vi "Main.vi"() -> ()   [LabVIEW 2013]
doc: "This Continuous Measurement sample project is based on the Queued Message Handler template.\n\nThe Event Handling Loop generates messages based on user interface actions.\n\nThe Message Handling Loop processes messages generated by the Event Handling Loop, or by other messages. There are also Acquisition and Logging message handling loop subVIs, and a chart updating loop."
uses:
  Settings/Settings.ctl
  Logging/Logging Configuration.ctl
  Piezo/Hardware Configuration.ctl
  Capacitive/Hardware Configuration.ctl
  Acquisition/Hardware Configuration.ctl
  Acquisition/Counter Configuration.ctl
  ADC/ADC Configuration.ctl
  controls/UI Data.ctl
  controls/UI State.ctl
  support/Message Queue/Enqueue Message (Single).vi
  <vilib>/measure/madcrms.llb/Averaged DC-RMS for 1 Chan.vi
  <vilib>/Utility/error.llb/Error Cluster From Error Code.vi
  <vilib>/ErrorRing/Error Ring.xnode
  Acquisition/Acquisition.lvlib
  Logging/Logging.lvlib
  Settings/Settings.lvlib
  support/User Event - Stop/User Event - Stop.lvlib
  support/Message Queue/Message Queue.lvlib
  <vilib>/ptbypt/NI_PtbyPt.lvlib
  Piezo/Piezo.lvlib
  Feedback/Feedback.lvlib
  <vilib>/measure/NI_MAPro.lvlib
  XY/XY.lvlib
  support/Data Notifiers/Data Notifiers.lvlib
  Capacitive/Capacitive.lvlib
panel:
  in  "Feedback Settings":T1={"Setpoint (cnt)"=10.0, "Refresh Time (s)"=1.0, "K_p (nm/cnt)"=0.3, "Averaging Time"=1.0, "T_i (s)"=0.3, "T_d (s)"=1.0, "Error Signal Source"=0} {"Error Signal Source" items=["External Input", "APD Signal"]}
  in  "Scan!":bool
  in  "Auto \nFB On":bool
  out "Control Status":string
  in  "Averaging Time (s)":dbl=3.0
  in  "Average and send\nto Setpoint":bool
  out "average":dbl
  in  "averaging time":dbl=1000.0 format="%#_13g"
  out "Cap Readout":sgl
  out "Cap Status":string
  in  "Enable Sensor":bool
  out "Status 4":string
  in  "initialize":bool
  in  "PSD points":i32=1000
  out "Status 3":string
  out "Y":sgl
  out "X":sgl
  in  "Next Button":bool
  in  "Up Button":bool
  in  "Down Button":bool
  in  "Previous Button":bool
  in  "Jog Speed":u16(ring) items=["0", "1", "2", "3"]
  in  "Enable XY":bool
  out "Status":bool
  in  "Settings 3":bool
  in  "Stop 2":bool
  in  "Start 2":bool
  in  "Settings 2":bool
  in  "Enable Feedback!":bool
  in  "Scan Settings":T2={"Dwell Time (s)"=1.0, "Max Height"=10.0, "Min Height"=9.0, "Step Size (um)"=0.01}
  in  "Start Saving":bool
  out "PiezoPosition":sgl
  out "Lag!! (unconnected)":bool
  out "Scan Duration: (s)":dbl
  in  "Do move":bool
  in  "Move to (um)":sgl
  out "PSD":dbl[](graph)
  out "Data":dbl[][](graph)
  in  "Settings":bool
  in  "Start":bool
  in  "Stop":bool
  out "Status":string
  in  "Exit":bool
  # "Recording"
  # "Position Control"
  # "Acquisition"
  # "Piezo Controller"
  # "X-Y Stage"
  # "Displacement Sensor"
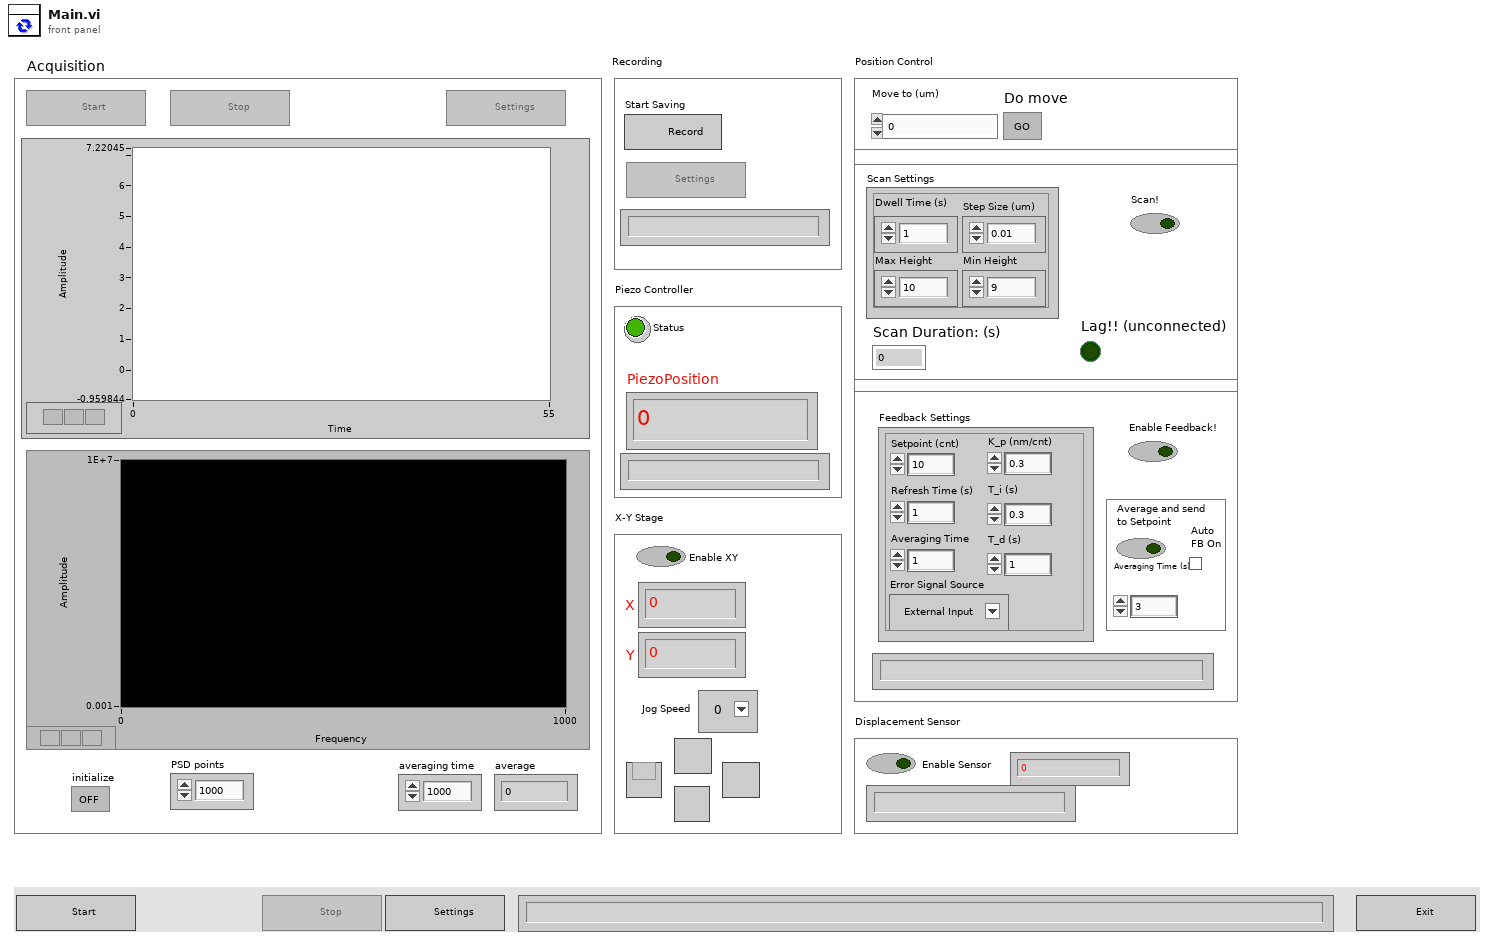
[diagram p1: front panel]
types:
  T1 = cluster{"Setpoint (cnt)":dbl, "Refresh Time (s)":dbl, "K_p (nm/cnt)":dbl, "Averaging Time":dbl, "T_i (s)":dbl, "T_d (s)":dbl, "Error Signal Source":u16}
  T2 = cluster{"Dwell Time (s)":dbl, "Max Height":dbl, "Min Height":dbl, "Step Size (um)":dbl}
  T3 = typedef "UI State.ctl" = cluster{"UI State":enum16{"Idle", "Acquiring and Logging", "Waiting for Exit", "Waiting for Stop"}, "Acq On":bool, "Log On":bool, "Piezo On":bool, "XY On":bool, "Cap On":bool}
  T4 = typedef "UI Data.ctl" = cluster{"Start Ref":refnum<vi>, "Trigger Ref":refnum<vi>, "Stop Ref":refnum<vi>, "Settings Ref":refnum<vi>, "Status Ref":refnum<vi>, "Exit Ref":refnum<vi>, "Data Ref":refnum<vi>, "Record Ref":refnum<vi>}
  T5 = typedef "Settings.lvlib/Settings.ctl" = cluster{"Logging Configuration":T6, "Piezo Config":T7, "Capacitive Config":T8, "Hardware Config":T9}
  T6 = typedef "Logging.lvlib/Logging Configuration.ctl" = cluster{"Log File Base Path":path, "Max Samples":u32, "File Refnum":refnum<file>, "Log Piezo":bool, "Piezo File Refnum":refnum<file>}
  T7 = typedef "Piezo.lvlib/Hardware Configuration.ctl" = cluster{"Piezo Serial Number":i32, "MG17Piezo":refnum<k7>, "Setpoint (um)":sgl}
  T8 = typedef "Capacitive.lvlib/Hardware Configuration.ctl" = cluster{"IP Address":string, "Handle":u32, "Refresh Time (ms)":dbl}
  T9 = typedef "Acquisition.lvlib/Hardware Configuration.ctl" = cluster{"Data Source":u16, "Counter Configuration":T10, "ADC Configuration":T11}
  T10 = typedef "Acquisition.lvlib/Counter Configuration.ctl" = cluster{"DAQmx Task":refnum<k21>, "Counter(s)":tag, "samples per readout":i32}
  T11 = typedef "Acquisition.lvlib/ADC Configuration.ctl" = cluster{"DAQmx Task":refnum<k21>, "Channel(s)":tag, "samples per readout":i32, "Sample Rate (s/s)":i32, "Max Voltage":dbl, "Min Voltage":dbl}
  T12 = typedef "Data Notifiers.lvlib/All Data Notifiers.ctl" = cluster{"APD Data Notifier":refnum<notifier>, "Piezo Readout Notifier":refnum<notifier>, "XY Readout Notifier":refnum<notifier>, "Capacitive Readout Notifier":refnum<notifier>}
  T13 = typedef "Message Queue.lvlib/All Message Queues.ctl" = cluster{"UI":refnum<queue>, "Acquisition":refnum<queue>, "Logging":refnum<queue>, "Piezo":refnum<queue>, "Feedback":refnum<queue>, "XY":refnum<queue>, "Capacitive":refnum<queue>}
  T14 = enum16{"Idle", "Acquiring and Logging", "Waiting for Exit", "Waiting for Stop"}
  T15 = enum8{"Enabled", "Disabled", "Disabled and Grayed Out"}
  T16 = typedef "Acquisition.lvlib/APD Notifier Cluster.ctl" = cluster{"data":dbl[][], "t0":i32}
  T17 = typedef "XY.lvlib/XY Display.ctl" = cluster{"X Position":sgl, "Y Position":sgl}
  T18 = typedef "Piezo.lvlib/Piezo display.ctl" = cluster{"PiezoPosition":sgl, "Counter Time":i32}
  T19 = typedef "Capacitive.lvlib/Capacitive Signal Cluster.ctl" = cluster{"Readout":sgl, "Time":i32}
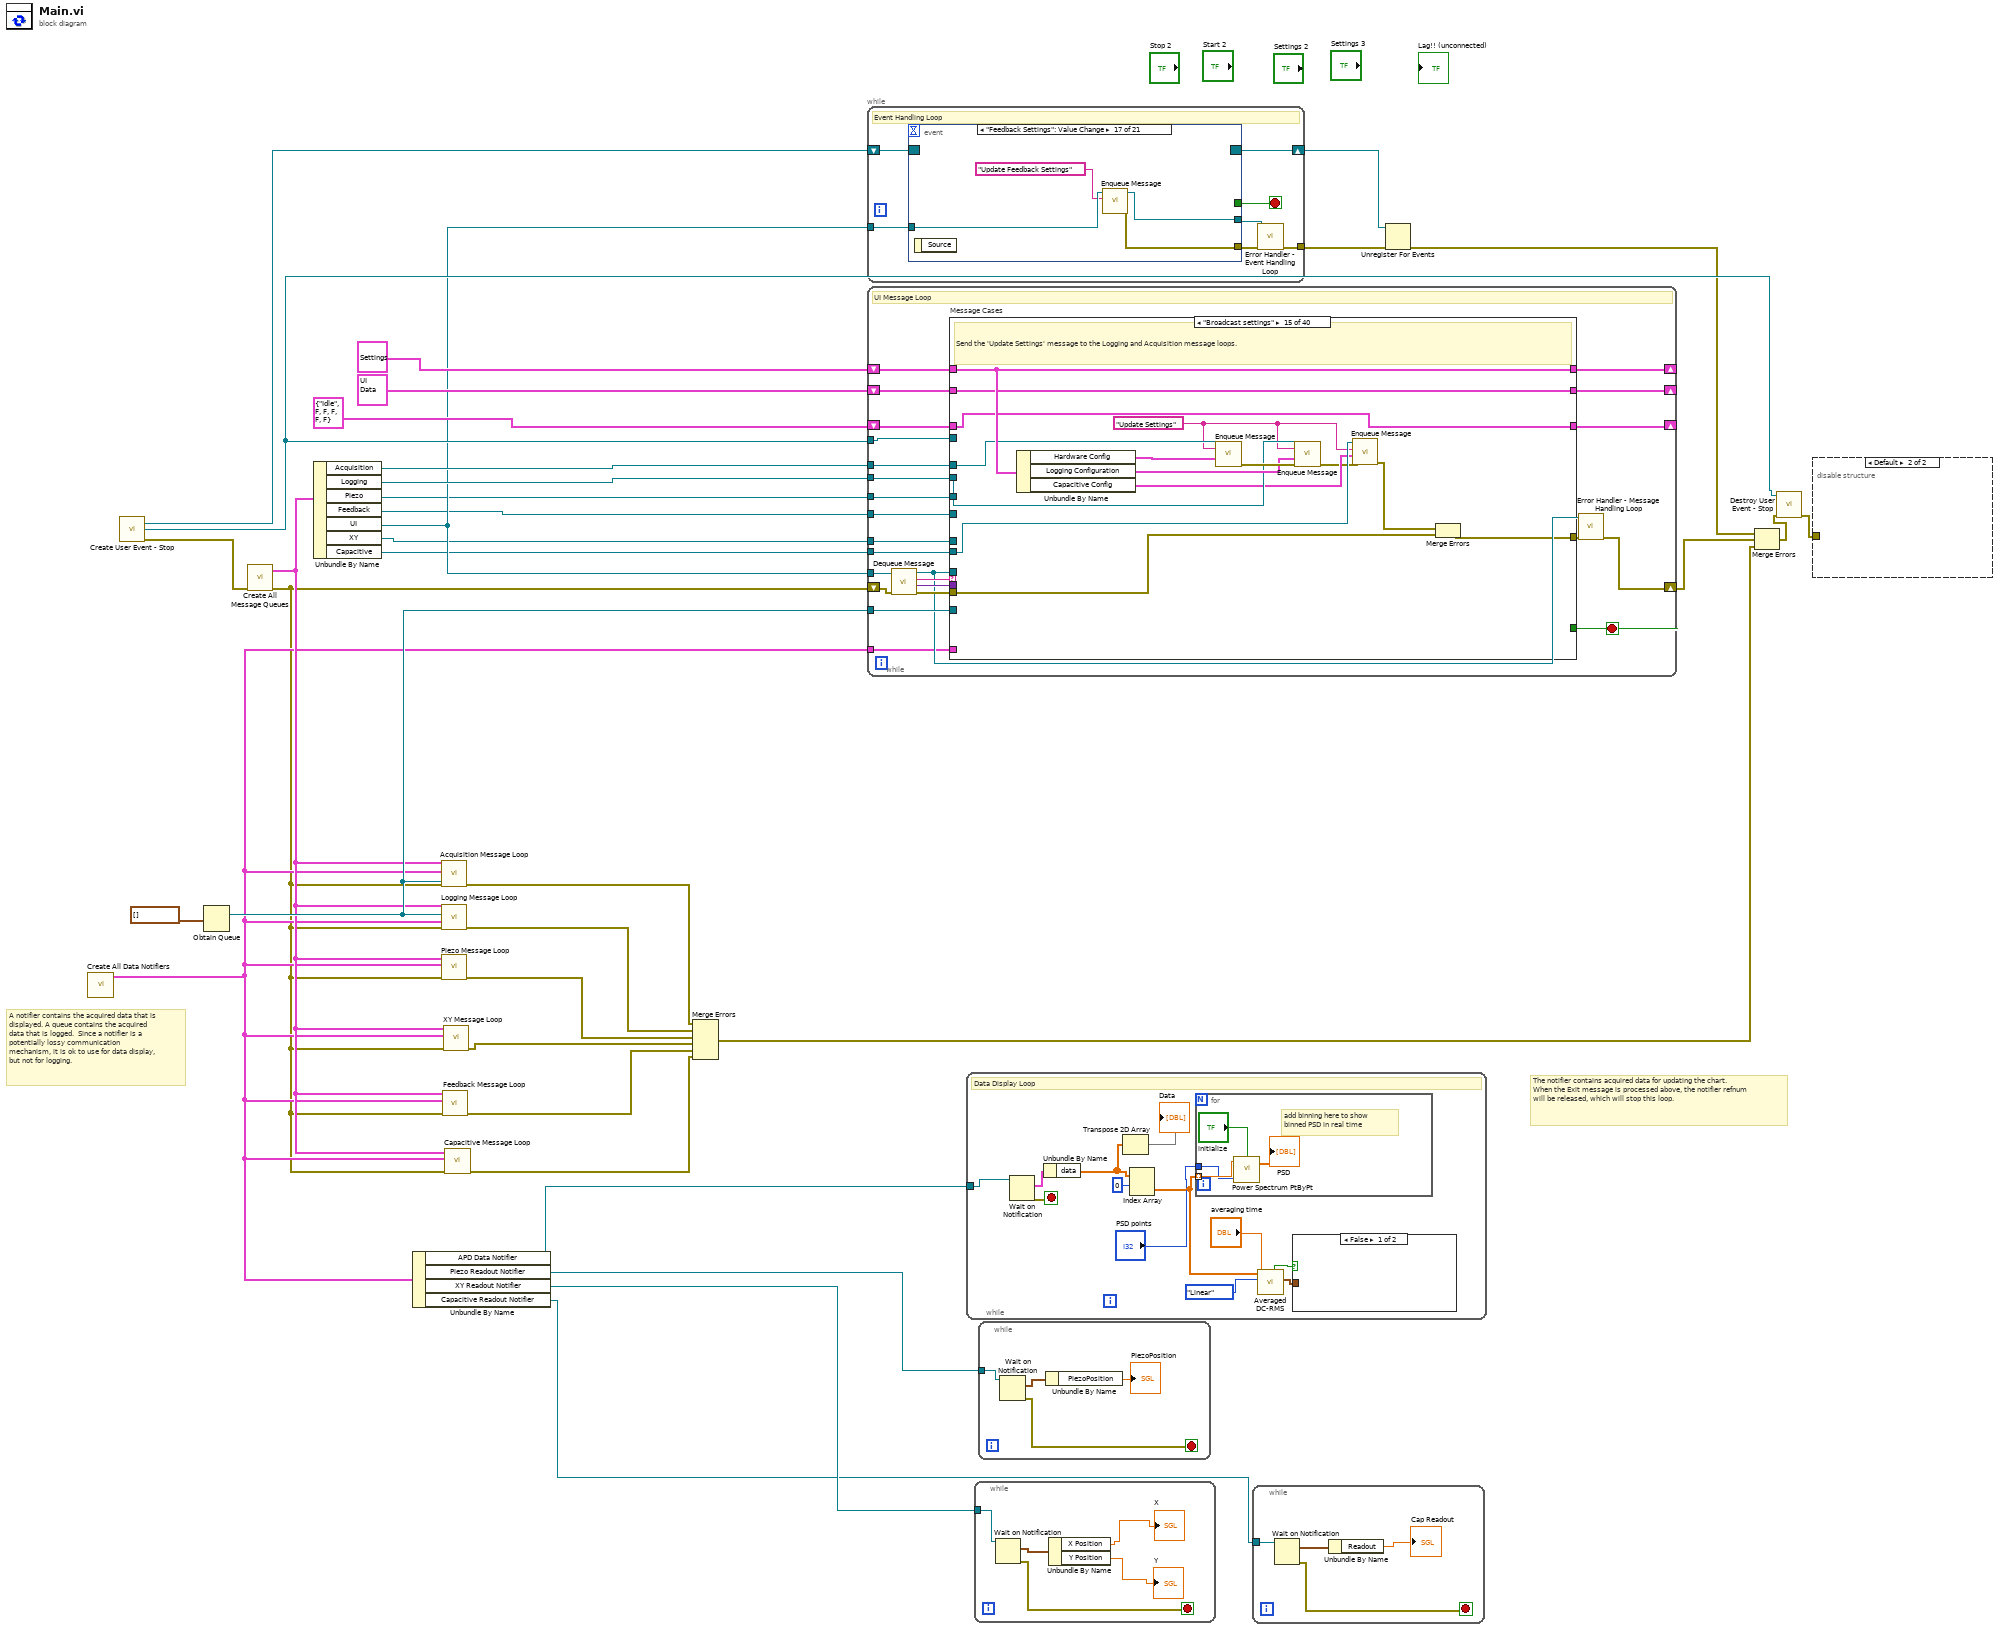
[diagram p0: block diagram]
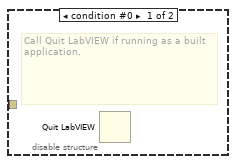
[diagram p2: hidden frame]
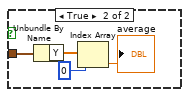
[diagram p3: hidden frame]
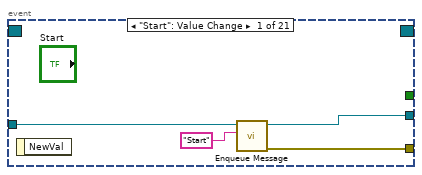
[diagram p4: hidden frame]
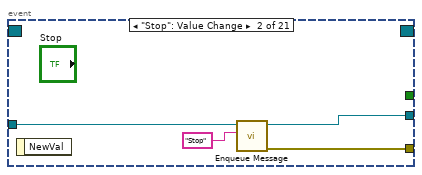
[diagram p5: hidden frame]
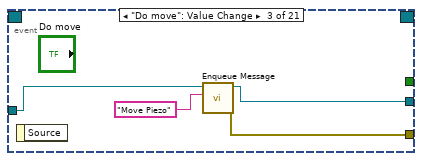
[diagram p6: hidden frame]
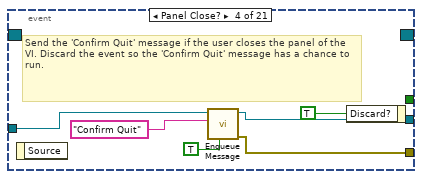
[diagram p7: hidden frame]
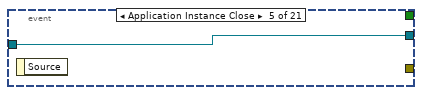
[diagram p8: hidden frame]
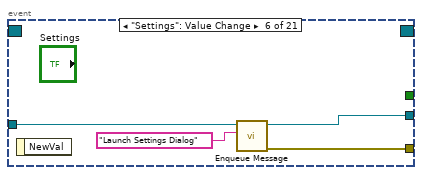
[diagram p9: hidden frame]
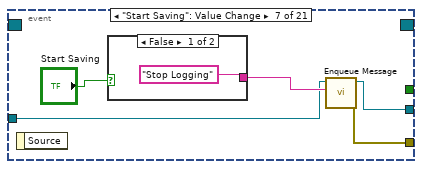
[diagram p10: hidden frame]
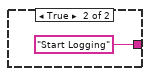
[diagram p11: hidden frame]
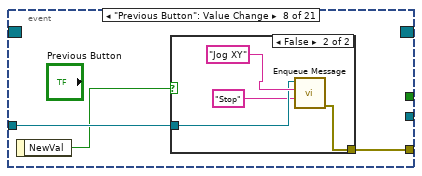
[diagram p12: hidden frame]
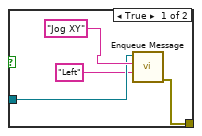
[diagram p13: hidden frame]
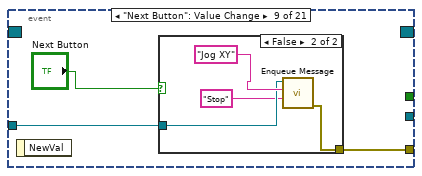
[diagram p14: hidden frame]
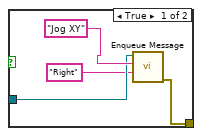
[diagram p15: hidden frame]
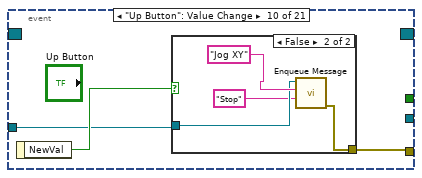
[diagram p16: hidden frame]
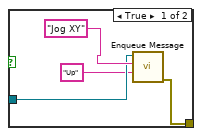
[diagram p17: hidden frame]
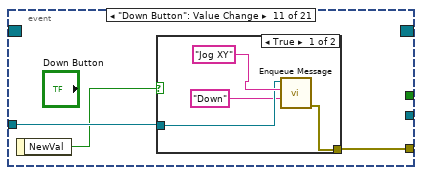
[diagram p18: hidden frame]
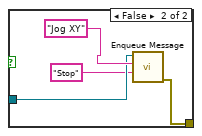
[diagram p19: hidden frame]
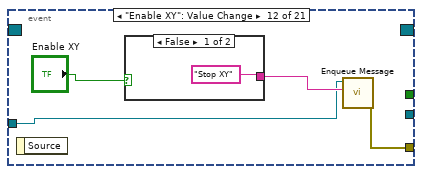
[diagram p20: hidden frame]
diagram:
  # "A notifier contains the acquired data that is displayed. A queue contains the acquired data that is logged.  Since a notifier is a potentially lossy communication mechanism, it is ok to use for data display, but not for logging."
  # "The notifier contains acquired data for updating the chart. When the Exit message is processed above, the notifier refnum will be released, which will stop this loop."
  n1 = call "Create All Data Notifiers.vi"() -> ("Initialized Data Notifiers"=w10:T12)  [unwired: 11 in]
  n2 = call "Create User Event - Stop.vi"() -> ("error out"=w30:errorcluster, "User Event - Stop"=w31:refnum<user-event>, "Stop Event Registration Refnum"=w32:refnum<event-registration>)  [unwired: 9 in]
  n3 = Obtain Queue(element data type=waveform(dbl)[] []) -> (queue out=w22:refnum<queue>)  [unwired: 4 in, 2 out]
  n4 = call "Create All Message Queues.vi"("error in (no error)"=w30) -> ("error out"=w9:errorcluster, "Message Queues out"=w11:T13)  [unwired: 9 in]
  n5 = Unbundle By Name(w11) -> ("Acquisition"=w25:refnum<queue>, "Logging"=w24:refnum<queue>, "Piezo"=w18:refnum<queue>, "Feedback"=w17:refnum<queue>, "UI"=w19:refnum<queue>, "XY"=w16:refnum<queue>, "Capacitive"=w12:refnum<queue>)
  n6 = Unbundle By Name(w10) -> ("APD Data Notifier"=w15:refnum<notifier>, "Piezo Readout Notifier"=w14:refnum<notifier>, "XY Readout Notifier"=w13:refnum<notifier>, "Capacitive Readout Notifier"=w1:refnum<notifier>)
  n7 = call "Acquisition Message Loop.vi"("error in (no error)"=w9, "Data Queue"=w22, "Data Notifiers"=w10, "Message Queues"=w11) -> ("error out"=w5:errorcluster)  [unwired: 7 in]
  n8 = call "Logging Message Loop.vi"("error in (no error)"=w9, "Data Notifiers"=w10, "Data Queue"=w22, "Message Queues"=w11) -> ("error out"=w6:errorcluster)  [unwired: 7 in]
  n9 = call "Piezo Message Loop.vi"("error in (no error)"=w9, "Data Notifiers"=w10, "Message Queues"=w11) -> ("error out"=w7:errorcluster)  [unwired: 8 in]
  n10 = call "Feedback Message Loop.vi"("error in (no error)"=w9, "Data Notifiers"=w10, "Message Queues"=w11) -> ("error out"=w4:errorcluster)  [unwired: 8 in]
  n11 = call "XY Message Loop.vi"("error in (no error)"=w9, "Data Notifiers"=w10, "Message Queues"=w11) -> ("error out"=w8:errorcluster)  [unwired: 8 in]
  n12 = call "Capacitive Message Loop.vi"("error in (no error)"=w9, "Data Notifiers"=w10, "Message Queues"=w11) -> ("error out"=w3:errorcluster)  [unwired: 8 in]
  n13 = Merge Errors(w5, w6, w7, w8, w4, w3) -> (w2:errorcluster)
  n14 = while {
    tunnel: w19 -> [w41]
    tunnel: [w36] -> w34
    shift-right: [w40] -> w27
    shift-left: w32 -> [w42]
    stop <- w39 stop-if-true
    # "Event Handling Loop"
    n15 = event shown="[16] \"Feedback Settings\": Value Change" {
      selector: w42 -> [_ _ _ _ _ _ _ _ _ _ _ _ _ _ _ _ _ _ _ _ _]
      dyn-events: [_ _ _ _ _ _ _ _ _ _ _ _ _ _ _ _ _ _ _ _ _] -> w40
      timeout: _ -> [_ _ _ _ _ _ _ _ _ _ _ _ _ _ _ _ _ _ _ _ _]
      tunnel: [_ _ _ _ _ _ _ _ _ _ _ _ _ _ _ _ _ _ _ TRUE ("Discard?") _] -> w39
      tunnel: w41 -> [w44 w49 w53 w60 w61 w63 w68 w75 w86 w96 w108 w119 w125 w130 w136 w144 w153 w158 w163 w167 _]
      tunnel: [w46 w48 w51 w55 _ w65 w67 w74 w85 w95 w106 w118 w124 w129 w135 w143 w150 w157 w166 _ _] -> w37
      tunnel: [w43 w47 w52 w56 w61 w62 w66 _ _ _ _ _ _ _ w133 w142 w151 w156 w162 w167 _] -> w38
      event "Start": Value Change {
        n16 = event-data() -> ()  [unwired: 1 in, 1 out]
        n17 = call-poly "Enqueue Message.vi"("Message"="Start", "Message Queue"=w44) -> ("error out"=w46:errorcluster, "dup Message Queue"=w43:refnum<queue>)  [unwired: 8 in]
      }
      event "Stop": Value Change {
        n18 = event-data() -> ()  [unwired: 1 in, 1 out]
        n19 = call-poly "Enqueue Message.vi"("Message"="Stop", "Message Queue"=w49) -> ("error out"=w48:errorcluster, "dup Message Queue"=w47:refnum<queue>)  [unwired: 8 in]
      }
      event "Do move": Value Change {
        n20 = event-data() -> ()  [unwired: 1 in, 1 out]
        n21 = call-poly "Enqueue Message.vi"("Message"="Move Piezo", "Message Queue"=w53) -> ("error out"=w51:errorcluster, "dup Message Queue"=w52:refnum<queue>)  [unwired: 8 in]
      }
      event Panel Close? {
        # "Send the 'Confirm Quit' message if the user closes the panel of the VI. Discard the event so the 'Confirm Quit' message has a chance to run."
        n22 = event-data() -> ()  [unwired: 1 in, 1 out]
        n23 = call-poly "Enqueue Message.vi"("Priority Message? (F)"=TRUE, "Message"="Confirm Quit", "Message Queue"=w60) -> ("error out"=w55:errorcluster, "dup Message Queue"=w56:refnum<queue>)  [unwired: 7 in]
        n24 = event-data("Discard?"=TRUE) -> ()  [unwired: 1 in, 1 out]
      }
      event Application Instance Close {
        n25 = event-data() -> ()  [unwired: 1 in, 1 out]
      }
      event "Settings": Value Change {
        n26 = event-data() -> ()  [unwired: 1 in, 1 out]
        n27 = call-poly "Enqueue Message.vi"("Message"="Launch Settings Dialog", "Message Queue"=w63) -> ("error out"=w65:errorcluster, "dup Message Queue"=w62:refnum<queue>)  [unwired: 8 in]
      }
      event "Start Saving": Value Change {
        n28 = event-data() -> ()  [unwired: 1 in, 1 out]
        n29 = case shown="False" "Start Saving" {
          tunnel: ["Stop Logging" ("Message") "Start Logging" ("Message")] -> w69
          frame False {
          }
          frame True {
          }
        }
        n30 = call-poly "Enqueue Message.vi"("Message"=w69, "Message Queue"=w68) -> ("error out"=w67:errorcluster, "dup Message Queue"=w66:refnum<queue>)  [unwired: 8 in]
      }
      event "Previous Button": Value Change {
        n31 = event-data() -> ("NewVal"=w73:bool)  [unwired: 1 in]
        n32 = case shown="False" w73 {
          tunnel: w75 -> [w78 w82]
          tunnel: [w76 w80] -> w74
          frame True {
            n33 = call-poly "Enqueue Message.vi"("Message Data"="Left" ("Message"), "Message"="Jog XY", "Message Queue"=w78) -> ("error out"=w76:errorcluster)  [unwired: 7 in, 1 out]
          }
          frame False {
            n34 = call-poly "Enqueue Message.vi"("Message Data"="Stop" ("Message"), "Message"="Jog XY", "Message Queue"=w82) -> ("error out"=w80:errorcluster)  [unwired: 7 in, 1 out]
          }
        }
      }
      event "Next Button": Value Change {
        n35 = event-data() -> ()  [unwired: 1 in, 1 out]
        n36 = case shown="False" "Next Button" {
          tunnel: w86 -> [w89 w93]
          tunnel: [w87 w91] -> w85
          frame True {
            n37 = call-poly "Enqueue Message.vi"("Message Data"="Right" ("Message"), "Message"="Jog XY", "Message Queue"=w89) -> ("error out"=w87:errorcluster)  [unwired: 7 in, 1 out]
          }
          frame False {
            n38 = call-poly "Enqueue Message.vi"("Message Data"="Stop" ("Message"), "Message"="Jog XY", "Message Queue"=w93) -> ("error out"=w91:errorcluster)  [unwired: 7 in, 1 out]
          }
        }
      }
      event "Up Button": Value Change {
        n39 = event-data() -> ("NewVal"=w97:bool)  [unwired: 1 in]
        n40 = case shown="False" w97 {
          tunnel: w96 -> [w100 w104]
          tunnel: [w98 w102] -> w95
          frame True {
            n41 = call-poly "Enqueue Message.vi"("Message Data"="Up" ("Message"), "Message"="Jog XY", "Message Queue"=w100) -> ("error out"=w98:errorcluster)  [unwired: 7 in, 1 out]
          }
          frame False {
            n42 = call-poly "Enqueue Message.vi"("Message Data"="Stop" ("Message"), "Message"="Jog XY", "Message Queue"=w104) -> ("error out"=w102:errorcluster)  [unwired: 7 in, 1 out]
          }
        }
      }
      event "Down Button": Value Change {
        n43 = event-data() -> ("NewVal"=w107:bool)  [unwired: 1 in]
        n44 = case shown="True" w107 {
          tunnel: w108 -> [w111 w115]
          tunnel: [w109 w113] -> w106
          frame True {
            n45 = call-poly "Enqueue Message.vi"("Message Data"="Down" ("Message"), "Message"="Jog XY", "Message Queue"=w111) -> ("error out"=w109:errorcluster)  [unwired: 7 in, 1 out]
          }
          frame False {
            n46 = call-poly "Enqueue Message.vi"("Message Data"="Stop" ("Message"), "Message"="Jog XY", "Message Queue"=w115) -> ("error out"=w113:errorcluster)  [unwired: 7 in, 1 out]
          }
        }
      }
      event "Enable XY": Value Change {
        n47 = event-data() -> ()  [unwired: 1 in, 1 out]
        n48 = case shown="False" "Enable XY" {
          tunnel: ["Stop XY" ("Message") "Start XY" ("Message")] -> w120
          frame False {
          }
          frame True {
          }
        }
        n49 = call-poly "Enqueue Message.vi"("Message"=w120, "Message Queue"=w119) -> ("error out"=w118:errorcluster)  [unwired: 8 in, 1 out]
      }
      event "Enable Sensor": Value Change {
        n50 = event-data() -> ()  [unwired: 1 in, 1 out]
        n51 = case shown="False" "Enable Sensor" {
          tunnel: ["Stop Cap" ("Message") "Start Cap" ("Message")] -> w126
          frame False {
          }
          frame True {
          }
        }
        n52 = call-poly "Enqueue Message.vi"("Message"=w126, "Message Queue"=w125) -> ("error out"=w124:errorcluster)  [unwired: 8 in, 1 out]
      }
      event "Jog Speed": Value Change {
        n53 = event-data() -> ()  [unwired: 1 in, 1 out]
        n54 = call-poly "Enqueue Message.vi"("Message Data"="Jog Speed", "Message"="Jog Speed", "Message Queue"=w130) -> ("error out"=w129:errorcluster)  [unwired: 7 in, 1 out]
      }
      event "Enable Feedback!": Value Change {
        n55 = event-data() -> ()  [unwired: 1 in, 1 out]
        n56 = case shown="False" "Enable Feedback!" {
          tunnel: ["Stop Feedback" ("Message") "Start Feedback" ("Message")] -> w137
          frame False {
          }
          frame True {
          }
        }
        n57 = call-poly "Enqueue Message.vi"("Message"=w137, "Message Queue"=w136) -> ("error out"=w135:errorcluster, "dup Message Queue"=w133:refnum<queue>)  [unwired: 8 in]
      }
      event "Scan!": Value Change {
        n58 = event-data() -> ()  [unwired: 1 in, 1 out]
        n59 = case shown="False" "Scan!" {
          tunnel: ["Stop Piezo Scan" ("Message") "Start Piezo Scan" ("Message")] -> w145
          tunnel: [FALSE ("Priority Message? (F)") FALSE ("Priority Message? (F)")] -> w140
          frame False {
          }
          frame True {
          }
        }
        n60 = call-poly "Enqueue Message.vi"("Priority Message? (F)"=w140, "Message"=w145, "Message Queue"=w144) -> ("error out"=w143:errorcluster, "dup Message Queue"=w142:refnum<queue>)  [unwired: 7 in]
      }
      event "Feedback Settings": Value Change {
        n61 = event-data() -> ()  [unwired: 1 in, 1 out]
        n62 = call-poly "Enqueue Message.vi"("Message"="Update Feedback Settings", "Message Queue"=w153) -> ("error out"=w150:errorcluster, "dup Message Queue"=w151:refnum<queue>)  [unwired: 8 in]
      }
      event "Average and send\nto Setpoint": Value Change {
        n63 = event-data() -> ()  [unwired: 1 in, 1 out]
        n64 = case shown="False" "Average and send\nto Setpoint" {
          tunnel: ["Stop Average and set" ("Message") "Start Average and set" ("Message")] -> w159
          frame False {
          }
          frame True {
          }
        }
        n65 = call-poly "Enqueue Message.vi"("Message Data"="Averaging Time (s)", "Message"=w159, "Message Queue"=w158) -> ("error out"=w157:errorcluster, "dup Message Queue"=w156:refnum<queue>)  [unwired: 7 in]
      }
      event "Exit": Value Change; Panel Close {
        w164 = TRUE  # Priority Message
        # "The UI Message Loop handles sending the Exit message to other loops."
        n66 = event-data() -> ()  [unwired: 1 in, 1 out]
        n67 = call-poly "Enqueue Message.vi"("Priority Message? (F)"=w164, "Message"="Exit", "Message Queue"=w163) -> ("error out"=w166:errorcluster, "dup Message Queue"=w162:refnum<queue>)  [unwired: 7 in]
      }
      event User Event {
        # "The Message Handling Loop processed an \"Exit\" message, which fired this event to stop the Event Handling Loop."
        n68 = event-data() -> ()  [unwired: 1 in, 1 out]
        n69 = local write "Status"("Exit" ("Exit String")) -> ()
      }
      event "Scan Settings": Value Change {
        n70 = event-data() -> ()  [unwired: 1 in, 1 out]
        n71 = local read "Scan Settings"() -> (w178:T2)
        n72 = Unbundle By Name(w178) -> ("Dwell Time (s)"=w171:dbl, "Max Height"=w177:dbl, "Min Height"=w176:dbl, "Step Size (um)"=w174:dbl)
        n73 = Subtract(x=w177, y=w176) -> (x-y=w175:dbl)
        n74 = Divide(x=w175, y=w174) -> (x/y=w173:dbl)
        n75 = Round Toward -Infinity(1:w173) -> (0:w172:dbl)
        n76 = Multiply(x=w171, y=w172) -> (x*y=→"Scan Duration: (s)":dbl)
      }
    }
    n77 = call "Error Handler - Event Handling Loop.vi"("error in (no error)"=w37, "Message Queue"=w38) -> ("dup error in"=w36:errorcluster)  [unwired: 8 in, 1 out]
  }
  n78 = while {
    tunnel: w19 -> [w196]
    tunnel: w31 -> [w201]
    shift-right: [w187] -> w35
    shift-left: w9 -> [w200]
    shift-right: [w195] -> _
    shift-left: T5 {"Logging Configuration"={"Log File Base Path"=path "", "Max Samples"=0, "File Refnum"=refnum, "Log Piezo"=FALSE, "Piezo File Refnum"=refnum}, "Piezo Config"={"Piezo Serial Number"=0, "MG17Piezo"=refnum, "Setpoint (um)"=0.0}, "Capacitive Config"={"IP Address"="", "Handle"=0, "Refresh Time (ms)"=0.0}, "Hardware Config"={"Data Source"=0, "Counter Configuration"={"DAQmx Task"="", "Counter(s)"="", "samples per readout"=0}, "ADC Configuration"={"DAQmx Task"="", "Channel(s)"="", "samples per readout"=0, "Sample Rate (s/s)"=0, "Max Voltage"=0.0, "Min Voltage"=0.0}}} ("Settings") -> [w194]
    shift-right: [w192] -> _
    shift-left: T4 {"Start Ref"=refnum, "Trigger Ref"=refnum, "Stop Ref"=refnum, "Settings Ref"=refnum, "Status Ref"=refnum, "Exit Ref"=refnum, "Data Ref"=refnum, "Record Ref"=refnum} ("Measurement UI Controls") -> [w193]
    tunnel: w25 -> [w191]
    tunnel: w24 -> [w190]
    tunnel: w22 -> [w189]
    shift-right: [w184] -> _
    shift-left: T3 {"UI State"=enum."Idle", "Acq On"=FALSE, "Log On"=FALSE, "Piezo On"=FALSE, "XY On"=FALSE, "Cap On"=FALSE} ("UI State") -> [w185]
    tunnel: w18 -> [w183]
    tunnel: w17 -> [w182]
    tunnel: w16 -> [w181]
    tunnel: w10 -> [w180]
    tunnel: w12 -> [w179]
    stop <- w202 stop-if-true
    # "UI Message Loop"
    n79 = call "Dequeue Message.vi"("error in (no error)"=w200, "Message Queue"=w196) -> ("error out"=w199:errorcluster, "Message Data"=w197:variant, "Message"=w198:string, "dup Message Queue"=w186:refnum<queue>)  [unwired: 6 in]
    n80 = case "Message Cases" shown="\"Broadcast settings\"" w198 {
      selector: w198 -> [_ _ _ _ _ _ _ _ _ _ _ _ _ _ _ _ _ _ _ _ _ _ _ _ _ _ _ _ _ _ _ _ _ _ _ _ _ _ _ w797]
      tunnel: w186 -> [w207 _ _ _ _ _ _ w372 w405 w412 w434 w452 w471 w490 _ w527 w542 w554 w591 _ _ _ _ _ _ _ _ _ _ _ _ _ _ _ _ w747 w767 _ _ _]
      tunnel: w199 -> [w206 w234 w245 w259 w269 w280 w293 w371 w404 w410 w432 w450 w469 w488 w516 w529 w546 w553 w596 w606 w611 w618 w626 w635 w642 w657 w667 w675 w685 w693 w701 w710 w718 w726 w734 w749 w769 w781 w790 _]
      tunnel: [w213 w234 w246 w260 w270 w281 w294 w373 w374 w411 w433 w451 w470 w489 w521 w524 w537 w552 w597 w605 w610 w624 w632 w633 w648 w651 w673 w681 w690 w698 w707 w715 w723 w731 w739 w750 w770 w780 w789 w798] -> w188
      tunnel: [_ _ _ _ _ _ _ _ _ _ _ _ _ _ _ _ _ _ TRUE _ _ _ _ _ _ _ _ _ _ _ _ _ _ _ _ _ _ _ _ _] -> w202
      tunnel: w197 -> [_ _ w244 w258 w268 w279 w292 _ _ _ _ _ _ _ _ _ w545 _ _ _ _ _ _ w634 _ w656 _ _ _ _ _ _ _ _ _ _ _ w784 w791 _]
      tunnel: w201 -> [_ _ _ _ _ _ _ _ _ _ _ _ _ _ _ _ _ _ w595 _ _ _ _ _ _ _ _ _ _ _ _ _ _ _ _ _ _ _ _ _]
      tunnel: [w216 w233 w241 w255 w265 w276 w290 w370 w403 w418 w439 w458 w477 w496 w519 w526 w548 w556 w593 w604 w614 w623 w631 w640 w647 w660 w672 w680 w689 w697 w706 w714 w722 w730 w738 w752 w772 w787 w795 w800] -> w195
      tunnel: w194 -> [w217 w233 w241 w255 w265 w276 w290 w370 w403 w418 w439 w458 w477 w496 w519 w530 w548 w556 w593 w604 w614 w623 w631 w640 w647 w660 w672 w680 w689 w697 w706 w714 w722 w730 w738 w752 w772 w787 w795 w800]
      tunnel: w193 -> [w209 w232 w240 w254 w264 w275 w289 w367 w400 w417 w431 w457 w476 w495 w515 w523 w547 w555 w592 w603 w613 w622 w630 w639 w646 w659 w671 w679 w688 w696 w705 w713 w721 w729 w737 w751 w771 w786 w794 w799]
      tunnel: [w209 w231 w240 w254 w264 w275 w289 w367 w400 w417 w431 w457 w476 w495 w515 w523 w547 w555 w592 w603 w613 w622 w630 w639 w646 w659 w671 w679 w688 w696 w705 w713 w721 w729 w737 w751 w771 w786 w794 w799] -> w192
      tunnel: w191 -> [_ _ _ _ _ _ _ w359 w389 _ _ _ _ _ w514 _ _ _ w584 _ _ _ _ _ _ _ _ _ _ _ _ _ _ _ _ _ _ _ _ _]
      tunnel: w190 -> [_ _ _ _ _ _ _ _ w391 _ _ _ _ _ w513 _ _ _ w583 _ _ _ _ _ _ _ w668 w676 _ _ _ _ _ _ _ _ _ _ _ _]
      tunnel: w189 -> [_ _ _ _ _ _ _ _ _ _ _ _ _ _ _ _ _ _ w590 _ _ _ _ _ _ _ _ _ _ _ _ _ _ _ _ _ _ _ _ _]
      tunnel: w185 -> [_ _ w235 w252 w263 w274 w288 _ w383 w415 w437 w455 w474 w493 w512 w522 w536 w550 _ w602 w607 w621 w629 w638 w645 w658 w670 w678 w687 w695 w704 w712 w720 w728 w736 w748 w768 w782 w788 w796]
      tunnel: [T3 {"UI State"=enum."Idle", "Acq On"=FALSE, "Log On"=FALSE, "Piezo On"=FALSE, "XY On"=FALSE, "Cap On"=FALSE} ("UI State") T3 {"UI State"=enum."Idle", "Acq On"=FALSE, "Log On"=FALSE, "Piezo On"=FALSE, "XY On"=FALSE, "Cap On"=FALSE} ("UI State") w235 w252 w263 w274 w288 T3 {"UI State"=enum."Idle", "Acq On"=TRUE, "Log On"=TRUE, "Piezo On"=TRUE, "XY On"=FALSE, "Cap On"=FALSE} ("UI State") w385 w415 w437 w455 w474 w493 w512 w522 w536 w551 T3 {"UI State"=enum."Idle", "Acq On"=FALSE, "Log On"=FALSE, "Piezo On"=FALSE, "XY On"=FALSE, "Cap On"=FALSE} ("UI State") w602 w607 w621 w629 w638 w645 w658 w670 w678 w687 w695 w704 w712 w720 w728 w736 w748 w768 w782 w788 w796] -> w184
      tunnel: w183 -> [_ _ _ _ _ _ _ w355 w379 _ _ _ _ _ _ _ _ _ w582 _ _ _ _ _ _ _ _ _ _ _ _ _ _ _ _ _ _ _ _ _]
      tunnel: w182 -> [_ _ _ _ _ _ _ w350 _ _ _ _ _ _ _ _ _ _ w581 _ w609 w619 w627 w636 w643 _ _ _ w682 w691 w699 _ _ _ _ _ _ _ _ _]
      tunnel: w181 -> [_ _ _ _ _ _ _ _ w376 _ _ _ _ _ _ _ _ _ w580 _ _ _ _ _ _ _ _ _ _ _ _ w708 _ _ w732 _ _ w785 w792 _]
      tunnel: w180 -> [_ _ _ _ _ _ _ _ _ _ _ _ _ _ _ _ _ _ w587 _ _ _ _ _ _ _ _ _ _ _ _ _ _ _ _ _ _ _ _ _]
      tunnel: w179 -> [_ _ _ _ _ _ _ _ _ _ _ _ _ _ w511 _ _ _ w578 _ _ _ _ _ _ _ _ _ _ _ _ _ w716 w724 _ _ _ _ _ _]
      frame "Initialize" {
        # "Initialize - Get configuration settings, then message the UI to initialize, and broadcast the settings to the other message loops."
        n81 = call "Load Settings from XML.vi"("Settings in"=w217) -> ("Settings out"=w216:T5)  [unwired: 9 in, 1 out]
        n82 = call-poly "Enqueue Message.vi"("error in (no error)"=w206, "Message"="Init UI Refs", "Message Queue"=w207) -> ("error out"=w204:errorcluster, "dup Message Queue"=w205:refnum<queue>)  [unwired: 7 in]
        n83 = call-poly "Enqueue Message.vi"("error in (no error)"=w204, "Message"="Broadcast Settings", "Message Queue"=w205) -> ("error out"=w215:errorcluster, "dup Message Queue"=w214:refnum<queue>)  [unwired: 7 in]
        n84 = call-poly "Enqueue Message.vi"("error in (no error)"=w215, "Message Data"="Ready..." ("Ready..."), "Message"="Update Status", "Message Queue"=w214) -> ("error out"=w213:errorcluster)  [unwired: 6 in, 1 out]
      }
      frame "Init UI Refs" {
        # "Enable: Start, Exit, Settings\nDisable: Stop"
        # "Init UI Refs - Store control references for UI controls.  Also enable/disable controls appropriately."
        n85 = property class="VI"("Front Panel.Closeable"=TRUE ("Front Panel Window:Closeable")) -> ()  [unwired: 2 in, 2 out]
        n86 = control-ref of="Data"() -> (w227:refnum<vi>)
        n87 = control-ref of="Start"() -> (w226:refnum<vi>)
        n88 = control-ref of="Stop"() -> (w221:refnum<vi>)
        n89 = control-ref of="Settings"() -> (w223:refnum<vi>)
        n90 = control-ref of="Exit"() -> (w222:refnum<vi>)
        n91 = control-ref of="Status"() -> (w228:refnum<vi>)
        n92 = control-ref of="Start Saving"() -> (w218:refnum<vi>)
        n93 = Build Array(w222, w223, w226) -> (w225:refnum<vi>[])
        n94 = Bundle By Name(cluster=w232, "Start Ref"=w226, "Stop Ref"=w221, "Settings Ref"=w223, "Status Ref"=w228, "Exit Ref"=w222, "Data Ref"=w227, "Record Ref"=w218) -> (w231:T4)
        n95 = Build Array(w221) -> (w220:refnum<vi>[])
        n96 = call "Set Enable State on Multiple Controls.vi"("Enable?"=TRUE, "Controls"=w225) -> ()  [unwired: 10 in]
        n97 = call "Set Enable State on Multiple Controls.vi"("Enable?"=FALSE, "Controls"=w220) -> ()  [unwired: 10 in]
      }
      frame "Update Status" {
        # "Update Display - Convert the message data to a string to display in the Status indicator."
        n98 = Variant To Data(error in=w245, type="", Variant=w244) -> (data=w237:string, error out=w242:errorcluster)
        "Status" <- w237
        n99 = Unbundle By Name(w240) -> ("Trigger Ref"=w236:refnum<vi>, "Stop Ref"=w239:refnum<vi>)
        n100 = property class="Bool"(reference=w239) -> ("DisabledEnum"=w238:T15)  [unwired: 1 in, 2 out]
        n101 = case shown="\"Enabled\"" w238 {
          tunnel: w237 -> [w249 _]
          tunnel: w236 -> [w250 _]
          frame "Enabled" {
            # "Disable the Force Trigger only while we are logging."
            n102 = Build Array(w250) -> (w251:refnum<vi>[])
            n103 = Not Equal?(x="Logging" ("Logging"), y=w249) -> (x != y?=w247:bool)
            n104 = call "Set Enable State on Multiple Controls.vi"("Enable?"=w247, "Controls"=w251) -> ()  [unwired: 10 in]
          }
          frame "Disabled", Default {
          }
        }
        n105 = Merge Errors(w242) -> (w246:errorcluster)
      }
      frame "Log Status" {
        # "Update Display - Convert the message data to a string to display in the Status indicator."
        n106 = Variant To Data(error in=w259, type="", Variant=w258) -> (data=→"Status 3":string, error out=w256:errorcluster)
        n107 = Merge Errors(w256) -> (w260:errorcluster)
      }
      frame "Piezo Status" {
        # "Update Display - Convert the message data to a string to display in the Status indicator."
        n108 = Variant To Data(error in=w269, type="", Variant=w268) -> (data=w262:string, error out=w266:errorcluster)
        "Status 4" <- w262
        n109 = case shown="\"Stopped\", Default" w262 {
          tunnel: [FALSE TRUE ("Status")] -> w261
          frame "Stopped", Default {
          }
          frame "Connected" {
          }
        }
        "Status" <- w261
        n110 = Merge Errors(w266) -> (w270:errorcluster)
      }
      frame "Cap Status" {
        # "Update Display - Convert the message data to a string to display in the Status indicator."
        n111 = Variant To Data(error in=w280, type="", Variant=w279) -> (data=→"Cap Status":string, error out=w277:errorcluster)
        n112 = Merge Errors(w277) -> (w281:errorcluster)
      }
      frame "Feedback Status" {
        # "Update Display - Convert the message data to a string to display in the Status indicator."
        n113 = Variant To Data(error in=w293, type="", Variant=w292) -> (data=w287:string, error out=w286:errorcluster)
        "Control Status" <- w287
        n114 = control-ref of="Average and send\nto Setpoint"() -> (w282:refnum<vi>)
        n115 = control-ref of="Enable Feedback!"() -> (w284:refnum<vi>)
        n116 = control-ref of="Scan!"() -> (w283:refnum<vi>)
        n117 = case shown="\"Ready...\"" w287 {
          tunnel: w286 -> [w295 w301 w307 w313 w321 w330 w339 w342]
          tunnel: [w295 w296 w303 w309 w319 w329 w337 w347] -> w285
          tunnel: w284 -> [_ w300 _ w312 w320 w324 w338 w348]
          tunnel: w283 -> [_ w299 w306 _ w316 w326 w333 w344]
          tunnel: w282 -> [_ _ w302 w308 w314 w323 w332 w345]
          frame "False", Default {
          }
          frame "Averaging Started..." {
            w298 = T15."Disabled and Grayed Out" ("Disabled")
            # "Disable Scan and Feedback while averaging"
            n118 = property class="Bool (strict)"(reference=w300, error in=w301, "DisabledEnum"=w298) -> (error out=w297:errorcluster)  [unwired: 1 out]
            n119 = property class="Bool (strict)"(reference=w299, error in=w297, "DisabledEnum"=w298) -> (error out=w296:errorcluster)  [unwired: 1 out]
          }
          frame "Feedback Started..." {
            w305 = T15."Disabled and Grayed Out" ("Disabled")
            # "Disable Scan and Average while Feedback On"
            n120 = property class="Bool (strict)"(reference=w302, error in=w307, "DisabledEnum"=w305) -> (error out=w304:errorcluster)  [unwired: 1 out]
            n121 = property class="Bool (strict)"(reference=w306, error in=w304, "DisabledEnum"=w305) -> (error out=w303:errorcluster)  [unwired: 1 out]
          }
          frame "Scan Started..." {
            w311 = T15."Disabled and Grayed Out" ("Disabled")
            # "Disable Avg and Feedback while Scanning"
            n122 = property class="Bool (strict)"(reference=w312, error in=w313, "DisabledEnum"=w311) -> (error out=w310:errorcluster)  [unwired: 1 out]
            n123 = property class="Bool (strict)"(reference=w308, error in=w310, "DisabledEnum"=w311) -> (error out=w309:errorcluster)  [unwired: 1 out]
          }
          frame "Averaging stopped... Ready" {
            w315 = T15."Enabled" ("Disabled")
            # "Enable Scan and Feedback buttons once averaging stopped"
            n124 = property class="Bool (strict)"(reference=w314, error in=w321, "Value"=FALSE) -> (error out=w318:errorcluster)  [unwired: 1 out]
            n125 = property class="Bool (strict)"(reference=w316, error in=w318, "DisabledEnum"=w315) -> (error out=w317:errorcluster)  [unwired: 1 out]
            n126 = property class="Bool (strict)"(reference=w320, error in=w317, "DisabledEnum"=w315) -> (error out=w319:errorcluster)  [unwired: 1 out]
          }
          frame "Feedback Stopped... Ready" {
            w325 = T15."Enabled" ("Disabled")
            # "Enable Scan and Average buttons once Feedback stopped"
            n127 = property class="Bool (strict)"(reference=w324, error in=w330, "Value"=FALSE) -> (error out=w328:errorcluster)  [unwired: 1 out]
            n128 = property class="Bool (strict)"(reference=w326, error in=w328, "DisabledEnum"=w325) -> (error out=w327:errorcluster)  [unwired: 1 out]
            n129 = property class="Bool (strict)"(reference=w323, error in=w327, "DisabledEnum"=w325) -> (error out=w329:errorcluster)  [unwired: 1 out]
          }
          frame "Scan Stopped... Ready" {
            w334 = T15."Enabled" ("Disabled")
            # "Enable Scan and Feedback buttons once averaging stopped"
            n130 = property class="Bool (strict)"(reference=w333, error in=w339, "Value"=FALSE) -> (error out=w336:errorcluster)  [unwired: 1 out]
            n131 = property class="Bool (strict)"(reference=w332, error in=w336, "DisabledEnum"=w334) -> (error out=w335:errorcluster)  [unwired: 1 out]
            n132 = property class="Bool (strict)"(reference=w338, error in=w335, "DisabledEnum"=w334) -> (error out=w337:errorcluster)  [unwired: 1 out]
          }
          frame "Ready..." {
            w343 = T15."Enabled" ("Disabled")
            # "Make sure all are enabled at first, in case program crashed\nearlier"
            n133 = property class="Bool (strict)"(reference=w344, error in=w342, "DisabledEnum"=w343) -> (error out=w341:errorcluster)  [unwired: 1 out]
            n134 = property class="Bool (strict)"(reference=w345, error in=w341, "DisabledEnum"=w343) -> (error out=w346:errorcluster)  [unwired: 1 out]
            n135 = property class="Bool (strict)"(reference=w348, error in=w346, "DisabledEnum"=w343) -> (error out=w347:errorcluster)  [unwired: 1 out]
          }
        }
        n136 = Merge Errors(w285) -> (w294:errorcluster)
      }
      frame "Start" {
        w349 = "Start" ("Message")
        # "Message Acquisition and Logging loops to start"
        # "Enable: Stop\nDisable: Start, Exit, Settings"
        # "Start - Enable/Disable buttons appropriately for an acquisition that has started, and update status display."
        n137 = Unbundle By Name(w367) -> ("Trigger Ref"=w357:refnum<vi>, "Stop Ref"=w358:refnum<vi>, "Start Ref"=w362:refnum<vi>, "Exit Ref"=w361:refnum<vi>, "Settings Ref"=w360:refnum<vi>)
        n138 = call-poly "Enqueue Message.vi"("error in (no error)"=w371, "Message Data"="Started" ("Waiting for trigger"), "Message"="Update Status", "Message Queue"=w372) -> ("error out"=w354:errorcluster)  [unwired: 6 in, 1 out]
        n139 = Build Array(w362, w361, w360) -> (w365:refnum<vi>[])
        n140 = Build Array(w357, w358) -> (w364:refnum<vi>[])
        n141 = call "Set Enable State on Multiple Controls.vi"("Enable?"=TRUE, "Controls"=w364) -> ()  [unwired: 10 in]
        n142 = call "Set Enable State on Multiple Controls.vi"("Enable?"=FALSE, "Controls"=w365) -> ()  [unwired: 10 in]
        n143 = call-poly "Enqueue Message.vi"("error in (no error)"=w354, "Message"=w349, "Message Queue"=w355) -> ("error out"=w353:errorcluster)  [unwired: 7 in, 1 out]
        n144 = call-poly "Enqueue Message.vi"("error in (no error)"=w353, "Message"=w349, "Message Queue"=w359) -> ("error out"=w352:errorcluster)  [unwired: 7 in, 1 out]
        n145 = call-poly "Enqueue Message.vi"("error in (no error)"=w352, "Message"=w349, "Message Queue"=w350) -> ("error out"=w351:errorcluster)  [unwired: 7 in, 1 out]
        n146 = Merge Errors(w351) -> (w373:errorcluster)
      }
      frame "Stop" {
        # "Message Acquisition and Logging loops to stop"
        # "Enable: Start, Exit, Settings\nDisable: Stop"
        # "Stop - Enable/Disable buttons appropriately for an acquisition that has stopped, and update status display."
        n147 = Unbundle By Name(w400) -> ("Trigger Ref"=w386:refnum<vi>, "Stop Ref"=w387:refnum<vi>, "Start Ref"=w395:refnum<vi>, "Exit Ref"=w394:refnum<vi>, "Settings Ref"=w393:refnum<vi>)
        n148 = Unbundle By Name(w383) -> ("UI State"=w384:T14)
        n149 = call-poly "Enqueue Message.vi"("error in (no error)"=w404, "Message Data"="Ready..." ("Ready..."), "Message"="Update Status", "Message Queue"=w405) -> ("error out"=w380:errorcluster)  [unwired: 6 in, 1 out]
        n150 = Build Array(w395, w394, w393) -> (w398:refnum<vi>[])
        n151 = Build Array(w386, w387) -> (w397:refnum<vi>[])
        n152 = call-poly "Enqueue Message.vi"("error in (no error)"=w380, "Message"="Stop", "Message Queue"=w379) -> ("error out"=w381:errorcluster)  [unwired: 7 in, 1 out]
        n153 = call "Set Enable State on Multiple Controls.vi"("Enable?"=FALSE, "Controls"=w397) -> ()  [unwired: 10 in]
        n154 = call "Set Enable State on Multiple Controls.vi"("Enable?"=TRUE, "Controls"=w398) -> ()  [unwired: 10 in]
        n155 = case shown="Default" w384 {
          tunnel: [w406 w409] -> w385
          tunnel: w383 -> [w407 w409]
          frame Default {
            n156 = Bundle By Name(cluster=w407, "UI State"=T14."Waiting for Stop") -> (w406:T3)
          }
          frame "Waiting for Exit" {
          }
        }
        n157 = call-poly "Enqueue Message.vi"("error in (no error)"=w381, "Message"="Stop", "Message Queue"=w391) -> ("error out"=w390:errorcluster)  [unwired: 7 in, 1 out]
        n158 = call-poly "Enqueue Message.vi"("error in (no error)"=w390, "Message"="Stop", "Message Queue"=w389) -> ("error out"=w377:errorcluster)  [unwired: 7 in, 1 out]
        n159 = call-poly "Enqueue Message.vi"("error in (no error)"=w377, "Message"="Stop", "Message Queue"=w376) -> ("error out"=w375:errorcluster)  [unwired: 7 in, 1 out]
        n160 = Merge Errors(w375) -> (w374:errorcluster)
      }
      frame "Acquisition Stopped" {
        # "Logic for determining what action to take when the acquisition has stopped."
        n161 = Bundle By Name(cluster=w415, "Acq On"=FALSE) -> (w414:T3)
        n162 = Unbundle By Name(w414) -> ("UI State"=w413:T14)
        n163 = case shown="\"Waiting for Exit\"" w413 {
          tunnel: w412 -> [_ _ w423 w428]
          tunnel: [w419 w420 w422 w426] -> w411
          tunnel: w410 -> [w419 w420 w421 w425]
          frame "Idle", Default {
          }
          frame "Acquiring and Logging" {
          }
          frame "Waiting for Exit" {
            n164 = call-poly "Enqueue Message.vi"("error in (no error)"=w421, "Message"="Verify Exit", "Message Queue"=w423) -> ("error out"=w422:errorcluster)  [unwired: 7 in, 1 out]
          }
          frame "Waiting for Stop" {
            n165 = call-poly "Enqueue Message.vi"("error in (no error)"=w425, "Message"="Verify Stop", "Message Queue"=w428) -> ("error out"=w426:errorcluster)  [unwired: 7 in, 1 out]
          }
        }
      }
      frame "Logging Stopped" {
        # "Logic for determining what action to take when the acquisition has stopped."
        n166 = Bundle By Name(cluster=w437, "Log On"=FALSE ("Acq On")) -> (w436:T3)
        n167 = Unbundle By Name(w436) -> ("UI State"=w435:T14)
        n168 = Unbundle By Name(w431) -> ("Record Ref"=w430:refnum<vi>)
        n169 = case shown="\"Acquiring and Logging\"" w435 {
          tunnel: w434 -> [_ _ w444 w449]
          tunnel: [w440 w441 w443 w447] -> w433
          tunnel: w432 -> [w440 w441 w442 w446]
          frame "Idle", Default {
          }
          frame "Acquiring and Logging" {
          }
          frame "Waiting for Exit" {
            n170 = call-poly "Enqueue Message.vi"("error in (no error)"=w442, "Message"="Verify Exit", "Message Queue"=w444) -> ("error out"=w443:errorcluster)  [unwired: 7 in, 1 out]
          }
          frame "Waiting for Stop" {
            n171 = call-poly "Enqueue Message.vi"("error in (no error)"=w446, "Message"="Verify Stop", "Message Queue"=w449) -> ("error out"=w447:errorcluster)  [unwired: 7 in, 1 out]
          }
        }
        n172 = property class="Bool"(reference=w430, "Value"=FALSE ("Start Saving")) -> ()  [unwired: 1 in, 2 out]
      }
      frame "Piezo Stopped" {
        # "Logic for determining what action to take when the acquisition has stopped."
        n173 = Bundle By Name(cluster=w455, "Piezo On"=FALSE ("Acq On")) -> (w454:T3)
        n174 = Unbundle By Name(w454) -> ("UI State"=w453:T14)
        n175 = case shown="\"Waiting for Exit\"" w453 {
          tunnel: w452 -> [_ _ w463 w468]
          tunnel: [w459 w460 w462 w466] -> w451
          tunnel: w450 -> [w459 w460 w461 w465]
          frame "Idle", Default {
          }
          frame "Acquiring and Logging" {
          }
          frame "Waiting for Exit" {
            n176 = call-poly "Enqueue Message.vi"("error in (no error)"=w461, "Message"="Verify Exit", "Message Queue"=w463) -> ("error out"=w462:errorcluster)  [unwired: 7 in, 1 out]
          }
          frame "Waiting for Stop" {
            n177 = call-poly "Enqueue Message.vi"("error in (no error)"=w465, "Message"="Verify Stop", "Message Queue"=w468) -> ("error out"=w466:errorcluster)  [unwired: 7 in, 1 out]
          }
        }
      }
      frame "XY Stopped" {
        # "Logic for determining what action to take when the acquisition has stopped."
        n178 = Bundle By Name(cluster=w474, "XY On"=FALSE ("Acq On")) -> (w473:T3)
        n179 = Unbundle By Name(w473) -> ("UI State"=w472:T14)
        n180 = case shown="\"Waiting for Stop\"" w472 {
          tunnel: w471 -> [_ _ w482 w487]
          tunnel: [w478 w479 w481 w485] -> w470
          tunnel: w469 -> [w478 w479 w480 w484]
          frame "Idle", Default {
          }
          frame "Acquiring and Logging" {
          }
          frame "Waiting for Exit" {
            n181 = call-poly "Enqueue Message.vi"("error in (no error)"=w480, "Message"="Verify Exit", "Message Queue"=w482) -> ("error out"=w481:errorcluster)  [unwired: 7 in, 1 out]
          }
          frame "Waiting for Stop" {
            n182 = call-poly "Enqueue Message.vi"("error in (no error)"=w484, "Message"="Verify Stop", "Message Queue"=w487) -> ("error out"=w485:errorcluster)  [unwired: 7 in, 1 out]
          }
        }
      }
      frame "Cap Stopped" {
        # "Logic for determining what action to take when the acquisition has stopped."
        n183 = Bundle By Name(cluster=w493, "Cap On"=FALSE ("Acq On")) -> (w492:T3)
        n184 = Unbundle By Name(w492) -> ("UI State"=w491:T14)
        n185 = case shown="\"Idle\", Default" w491 {
          tunnel: w490 -> [_ _ w501 w506]
          tunnel: [w497 w498 w500 w504] -> w489
          tunnel: w488 -> [w497 w498 w499 w503]
          frame "Idle", Default {
          }
          frame "Acquiring and Logging" {
          }
          frame "Waiting for Exit" {
            n186 = call-poly "Enqueue Message.vi"("error in (no error)"=w499, "Message"="Verify Exit", "Message Queue"=w501) -> ("error out"=w500:errorcluster)  [unwired: 7 in, 1 out]
          }
          frame "Waiting for Stop" {
            n187 = call-poly "Enqueue Message.vi"("error in (no error)"=w503, "Message"="Verify Stop", "Message Queue"=w506) -> ("error out"=w504:errorcluster)  [unwired: 7 in, 1 out]
          }
        }
      }
      frame "Broadcast settings" {
        w509 = "Update Settings" ("Message")
        # "Send the 'Update Settings' message to the Logging and Acquisition message loops."
        n188 = Unbundle By Name(w519) -> ("Hardware Config"=w518:T9, "Logging Configuration"=w517:T6, "Capacitive Config"=w510:T8)
        n189 = call-poly "Enqueue Message.vi"("Message Data"=w518, "Message"=w509, "Message Queue"=w514) -> ("error out"=w520:errorcluster)  [unwired: 7 in, 1 out]
        n190 = call-poly "Enqueue Message.vi"("error in (no error)"=w520, "Message Data"=w517, "Message"=w509, "Message Queue"=w513) -> ("error out"=w508:errorcluster)  [unwired: 6 in, 1 out]
        n191 = call-poly "Enqueue Message.vi"("error in (no error)"=w508, "Message Data"=w510, "Message"=w509, "Message Queue"=w511) -> ("error out"=w507:errorcluster)  [unwired: 6 in, 1 out]
        n192 = Merge Errors(w507, w516) -> (w521:errorcluster)
      }
      frame "Launch Settings Dialog" {
        # "Launch the Settings Dialog when the user clicks the 'Settings' button."
        n193 = call "Settings Dialog.vi"("error in (no error)"=w529, "Settings in"=w530) -> ("error out"=w525:errorcluster, "Cancelled?"=w528:bool, "Settings out"=w526:T5)  [unwired: 6 in, 1 out]
        n194 = case shown="False" w528 {
          tunnel: w527 -> [w534 _]
          tunnel: w525 -> [w533 w535]
          tunnel: [w532 w535] -> w524
          frame False {
            n195 = call-poly "Enqueue Message.vi"("error in (no error)"=w533, "Message"="Broadcast Settings", "Message Queue"=w534) -> ("error out"=w532:errorcluster)  [unwired: 7 in, 1 out]
          }
          frame True {
          }
        }
      }
      frame "Error" {
        # "Error - Check the error message data and respond accordingly. This message is sent by the \"Error Handler\" VIs at the end of each loop in this application."
        n196 = Variant To Data(error in=w546, type=errorcluster {"status"=FALSE, "code"=0, "source"=""} ("error out"), Variant=w545) -> (data=w543:errorcluster, error out=w539:errorcluster)
        n197 = call <vilib>:"Simple Error Handler.vi"("error in (no error)"=w543) -> ()  [unwired: 4 in, 5 out]
        n198 = call-poly "Enqueue Message.vi"("Priority Message? (F)"=TRUE, "Message"="Exit", "Message Queue"=w542) -> ("error out"=w538:errorcluster)  [unwired: 7 in, 1 out]
        n199 = Merge Errors(w538, w539) -> (w537:errorcluster)
      }
      frame "Confirm Quit" {
        # "Confirm Quit - Message that can confirm whether or not the user wants to exit the application."
        n200 = Unbundle By Name(w550) -> ("UI State"=w549:T14)
        n201 = case shown="Default" w549 {
          tunnel: w554 -> [w561 w567]
          tunnel: w553 -> [w560 w565]
          tunnel: [w557 w564] -> w552
          tunnel: [T3 {"UI State"=enum."Idle", "Acq On"=FALSE, "Log On"=FALSE, "Piezo On"=FALSE, "XY On"=FALSE, "Cap On"=FALSE} ("UI State") w563] -> w551
          frame Default {
            # "If 'Confirm Quit' comes in while the system is idle, there is no need for a confirmation message."
            n202 = call-poly "Enqueue Message.vi"("Priority Message? (F)"=TRUE, "error in (no error)"=w560, "Message"="Exit", "Message Queue"=w561) -> ("error out"=w557:errorcluster)  [unwired: 6 in, 1 out]
          }
          frame "Acquiring and Logging" {
            n203 = Two Button Dialog(message="Are you sure you want to quit while the acquisition is running?" ("Confirm Quit Message"), 1:"No" ("No"), 2:"Yes" ("Yes")) -> (T button?=w566:bool)
            n204 = case shown="True" w566 {
              tunnel: w567 -> [_ w577]
              tunnel: w565 -> [w571 w576]
              tunnel: [w571 w575] -> w564
              tunnel: [T3 {"UI State"=enum."Idle", "Acq On"=FALSE, "Log On"=FALSE, "Piezo On"=FALSE, "XY On"=FALSE, "Cap On"=FALSE} ("UI State") T3 {"UI State"=enum."Idle", "Acq On"=FALSE, "Log On"=FALSE, "Piezo On"=FALSE, "XY On"=FALSE, "Cap On"=FALSE} ("UI State")] -> w563
              frame False {
                # "User did not want to quit."
              }
              frame True {
                n205 = call-poly "Enqueue Message.vi"("error in (no error)"=w576, "Message"="Stop", "Message Queue"=w577) -> ("error out"=w575:errorcluster)  [unwired: 7 in, 1 out]
              }
            }
          }
        }
      }
      frame "Exit" {
        # "Don't check the error outs. The acquisition and logging queues may have already been released."
        # "Close references owned by the Main VI."
        # "Stop the VI"
        # "Exit - Fire the User Event to stop the Event Handling Loop.  Also send Exit messages to the Acquisition and Logging loops."
        n206 = Release Queue(queue=w591, error in (no error)=w596) -> (error out=w588:errorcluster)  [unwired: 1 in, 2 out]
        n207 = call "Fire User Event - Stop.vi"("User Event - Stop"=w595) -> ("error out"=w594:errorcluster)  [unwired: 10 in]
        n208 = Build Array(w584, w583, w582, w581, w580, w578) -> (w579:refnum<queue>[])
        n209 = Release Queue(queue=w590, error in (no error)=w588) -> (error out=w586:errorcluster)  [unwired: 1 in, 2 out]
        n210 = for {
          tunnel: w579 -> [w600] mode=indexing
          n211 = call-poly "Enqueue Message.vi"("Priority Message? (F)"=TRUE, "Message"="Exit", "Message Queue"=w600) -> ()  [unwired: 7 in, 2 out]
        }
        n212 = call "Release All Notifiers.vi"("error in (no error)"=w586, "All Data Notifiers"=w587) -> ("error out"=w585:errorcluster)  [unwired: 9 in]
        n213 = Merge Errors(w594, w585) -> (w597:errorcluster)
      }
      frame "---Copy This Frame---" {
        # "Duplicate this frame when creating new messages.  Change this comment in the duplicated frame to describe this message."
        n214 = Merge Errors(w606) -> (w605:errorcluster)
      }
      frame "Update Feedback Settings" {
        n215 = call-poly "Enqueue Message.vi"("error in (no error)"=w611, "Message Data"="Feedback Settings", "Message"="Update Feedback Settings", "Message Queue"=w609) -> ("error out"=w610:errorcluster)  [unwired: 6 in, 1 out]
      }
      frame "Start Feedback" {
        # "Tell Feedback Message Loop to go into feedback mode"
        n216 = control-ref of="Feedback Settings"() -> (w616:refnum<vi>)
        n217 = property class="Clust (strict)"(reference=w616) -> ("Value"=w615:T1)  [unwired: 1 in, 2 out]
        n218 = call-poly "Enqueue Message.vi"("error in (no error)"=w618, "Message Data"=w615, "Message"="Start Feedback", "Message Queue"=w619) -> ("error out"=w617:errorcluster)  [unwired: 6 in, 1 out]
        n219 = Merge Errors(w617) -> (w624:errorcluster)
      }
      frame "Stop Feedback" {
        # "Duplicate this frame when creating new messages.  Change this comment in the duplicated frame to describe this message."
        n220 = call-poly "Enqueue Message.vi"("error in (no error)"=w626, "Message"="Stop Feedback", "Message Queue"=w627) -> ("error out"=w625:errorcluster)  [unwired: 7 in, 1 out]
        n221 = Merge Errors(w625) -> (w632:errorcluster)
      }
      frame "Start Average and set" {
        # "Tell feedback loop to start averaging"
        # "Duplicate this frame when creating new messages.  Change this comment in the duplicated frame to describe this message."
        n222 = call-poly "Enqueue Message.vi"("error in (no error)"=w635, "Message Data"=w634, "Message"="Start Average and set", "Message Queue"=w636) -> ("error out"=w633:errorcluster)  [unwired: 6 in, 1 out]
      }
      frame "Stop Average and set" {
        # "Duplicate this frame when creating new messages.  Change this comment in the duplicated frame to describe this message."
        n223 = call-poly "Enqueue Message.vi"("error in (no error)"=w642, "Message"="Stop Average and set", "Message Queue"=w643) -> ("error out"=w641:errorcluster)  [unwired: 7 in, 1 out]
        n224 = Merge Errors(w641) -> (w648:errorcluster)
      }
      frame "Adjust Setpoint" {
        # "Change the value of 'SETPOINT'"
        # "Duplicate this frame when creating new messages.  Change this comment in the duplicated frame to describe this message."
        n225 = Variant To Data(error in=w657, type=0.0 ("Running average"), Variant=w656) -> (data=w654:dbl, error out=w653:errorcluster)
        n226 = control-ref of="Setpoint (cnt)"() -> (w649:refnum<vi>)
        n227 = property class="DigNum (strict)"(reference=w649, error in=w653, "Val(Sgnl)"=w654) -> (error out=w652:errorcluster)  [unwired: 1 out]
        n228 = case shown="False" "Auto \nFB On" {
          tunnel: w652 -> [w661 w664]
          tunnel: [w661 w663] -> w651
          frame False {
          }
          frame True {
            # "'Press' the Enable feedback button"
            n229 = control-ref of="Enable Feedback!"() -> (w662:refnum<vi>)
            n230 = property class="Bool (strict)"(reference=w662, error in=w664, "Val(Sgnl)"=TRUE ("Value (Signaling)")) -> (error out=w663:errorcluster)  [unwired: 1 out]
          }
        }
      }
      frame "Start Logging" {
        # "Start the logging loop"
        # "Duplicate this frame when creating new messages.  Change this comment in the duplicated frame to describe this message."
        n231 = call-poly "Enqueue Message.vi"("error in (no error)"=w667, "Message"="Start", "Message Queue"=w668) -> ("error out"=w666:errorcluster)  [unwired: 7 in, 1 out]
        n232 = Merge Errors(w666) -> (w673:errorcluster)
      }
      frame "Stop Logging" {
        # "Stop the logging loop"
        # "Duplicate this frame when creating new messages.  Change this comment in the duplicated frame to describe this message."
        n233 = call-poly "Enqueue Message.vi"("error in (no error)"=w675, "Message"="Stop", "Message Queue"=w676) -> ("error out"=w674:errorcluster)  [unwired: 7 in, 1 out]
        n234 = Merge Errors(w674) -> (w681:errorcluster)
      }
      frame "Start Piezo Scan" {
        # "Duplicate this frame when creating new messages.  Change this comment in the duplicated frame to describe this message."
        n235 = call-poly "Enqueue Message.vi"("error in (no error)"=w685, "Message Data"="Scan Settings", "Message"="Start Scan", "Message Queue"=w682) -> ("error out"=w684:errorcluster)  [unwired: 6 in, 1 out]
        n236 = Merge Errors(w684) -> (w690:errorcluster)
      }
      frame "Stop Piezo Scan" {
        # "Duplicate this frame when creating new messages.  Change this comment in the duplicated frame to describe this message."
        n237 = call-poly "Enqueue Message.vi"("error in (no error)"=w693, "Message"="Stop Scan", "Message Queue"=w691) -> ("error out"=w692:errorcluster)  [unwired: 7 in, 1 out]
        n238 = Merge Errors(w692) -> (w698:errorcluster)
      }
      frame "Move Piezo" {
        # "Duplicate this frame when creating new messages.  Change this comment in the duplicated frame to describe this message."
        n239 = call-poly "Enqueue Message.vi"("error in (no error)"=w701, "Message Data"="Move to (um)", "Message"="Go To", "Message Queue"=w699) -> ("error out"=w700:errorcluster)  [unwired: 6 in, 1 out]
        n240 = Merge Errors(w700) -> (w707:errorcluster)
      }
      frame "Start XY" {
        # "Duplicate this frame when creating new messages.  Change this comment in the duplicated frame to describe this message."
        n241 = call-poly "Enqueue Message.vi"("error in (no error)"=w710, "Message"="Start", "Message Queue"=w708) -> ("error out"=w709:errorcluster)  [unwired: 7 in, 1 out]
        n242 = Merge Errors(w709) -> (w715:errorcluster)
      }
      frame "Start Cap" {
        # "Duplicate this frame when creating new messages.  Change this comment in the duplicated frame to describe this message."
        n243 = call-poly "Enqueue Message.vi"("error in (no error)"=w718, "Message"="Start", "Message Queue"=w716) -> ("error out"=w717:errorcluster)  [unwired: 7 in, 1 out]
        n244 = Merge Errors(w717) -> (w723:errorcluster)
      }
      frame "Stop Cap" {
        # "Duplicate this frame when creating new messages.  Change this comment in the duplicated frame to describe this message."
        n245 = call-poly "Enqueue Message.vi"("error in (no error)"=w726, "Message"="Stop", "Message Queue"=w724) -> ("error out"=w725:errorcluster)  [unwired: 7 in, 1 out]
        n246 = Merge Errors(w725) -> (w731:errorcluster)
      }
      frame "Stop XY" {
        # "Duplicate this frame when creating new messages.  Change this comment in the duplicated frame to describe this message."
        n247 = call-poly "Enqueue Message.vi"("error in (no error)"=w734, "Message"="Stop", "Message Queue"=w732) -> ("error out"=w733:errorcluster)  [unwired: 7 in, 1 out]
        n248 = Merge Errors(w733) -> (w739:errorcluster)
      }
      frame "Verify Stop" {
        # "Duplicate this frame when creating new messages.  Change this comment in the duplicated frame to describe this message."
        n249 = Unbundle By Name(w748) -> ("Acq On"=w746:bool, "Log On"=w745:bool, "Piezo On"=w744:bool, "XY On"=w740:bool)
        n250 = Build Array(w746, w745, w744, w740) -> (w743:bool[])
        n251 = Or Array Elements(Boolean array=w743) -> (logical OR=w742:bool)
        n252 = Not(x=w742) -> (.not. x?=w741:bool)
        n253 = case shown="True" w741 {
          tunnel: [w753 w756] -> w750
          tunnel: w749 -> [w753 w755]
          tunnel: w747 -> [_ w754]
          frame False {
          }
          frame True {
            # "If everything is off, then update status."
            n254 = call-poly "Enqueue Message.vi"("error in (no error)"=w755, "Message Data"="Ready..." ("Message"), "Message"="Update Status", "Message Queue"=w754) -> ("error out"=w757:errorcluster)  [unwired: 6 in, 1 out]
            n255 = Merge Errors(w757) -> (w756:errorcluster)
          }
        }
      }
      frame "Verify Exit" {
        # "Duplicate this frame when creating new messages.  Change this comment in the duplicated frame to describe this message."
        n256 = Unbundle By Name(w768) -> ("Acq On"=w766:bool, "Log On"=w765:bool, "Piezo On"=w764:bool, "XY On"=w760:bool)
        n257 = Build Array(w766, w765, w764, w760) -> (w763:bool[])
        n258 = Or Array Elements(Boolean array=w763) -> (logical OR=w762:bool)
        n259 = Not(x=w762) -> (.not. x?=w761:bool)
        n260 = case shown="True" w761 {
          tunnel: [w773 w777] -> w770
          tunnel: w769 -> [w773 w776]
          tunnel: w767 -> [_ w775]
          frame False {
          }
          frame True {
            # "If everything is off, then exit."
            n261 = call-poly "Enqueue Message.vi"("Priority Message? (F)"=TRUE, "error in (no error)"=w776, "Message"="Exit", "Message Queue"=w775) -> ("error out"=w778:errorcluster)  [unwired: 6 in, 1 out]
            n262 = Merge Errors(w778) -> (w777:errorcluster)
          }
        }
      }
      frame "Jog XY" {
        n263 = call-poly "Enqueue Message.vi"("error in (no error)"=w781, "Message Data"=w784, "Message"="Jog", "Message Queue"=w785) -> ("error out"=w780:errorcluster)  [unwired: 6 in, 1 out]
      }
      frame "Jog Speed" {
        n264 = call-poly "Enqueue Message.vi"("error in (no error)"=w790, "Message Data"=w791, "Message"="Speed", "Message Queue"=w792) -> ("error out"=w789:errorcluster)  [unwired: 6 in, 1 out]
      }
      frame Default {
        # "'Default' case only runs if there is a message that isn't defined in any of the other cases.  Output a programming error."
        n265 = xnode "Error Ring"("parameter 0"=w797) -> ("error out"=w798:errorcluster)
      }
    }
    n266 = call "Error Handler - Message Handling Loop.vi"("error in (no error)"=w188, "Message Queue"=w186) -> ("dup error in"=w187:errorcluster)  [unwired: 8 in, 1 out]
  }
  n267 = while "Data Display Loop" {
    tunnel: w15 -> [w813]
    stop <- w819 stop-if-true
    # "Data Display Loop"
    n268 = Wait on Notification(notifier=w813) -> (notification=w812:T16, error out=w819:errorcluster)  [unwired: 3 in, 2 out]
    n269 = Unbundle By Name(w812) -> ("data"=w808:dbl[][])
    n270 = Transpose 2D Array(2D array=w808) -> (transposed array=→"Data":dbl[][])
    n271 = Index Array(array=w808, index (row)=0) -> (element=w811:dbl[])  [unwired: 1 in]
    n272 = for {
      tunnel: w811 -> [w827] mode=indexing
      tunnel: "PSD points" -> [w826]
      # "add binning here to show \nbinned PSD in real time"
      n273 = call <vilib>:"Power Spectrum PtByPt.vi"("initialize"="initialize", "sample length"=w826, "x"=w827) -> ("Power Spectrum"=→"PSD":dbl[])  [unwired: 1 in, 1 out]
    }
    n274 = call-poly <vilib>:"Averaged DC-RMS.vi"("averaging time"="averaging time", "averaging type"=enum16{"Linear", "Exponential"}."Linear", "signal in"=w811) -> ("RMS value waveform"=w816:waveform(dbl), "data ready"=w815:bool)  [unwired: 4 in, 3 out]
    n275 = case shown="False" w815 {
      tunnel: w816 -> [_ w823]
      frame False {
      }
      frame True {
        n276 = Unbundle By Name(w823) -> ("Y"=w822:dbl[])
        n277 = Index Array(array=w822, index=0) -> (element=→"average":dbl)
      }
    }
  }
  n278 = while {
    tunnel: w13 -> [w830]
    stop <- w831 stop-if-true
    n279 = Wait on Notification(notifier=w830) -> (notification=w832:T17, error out=w831:errorcluster)  [unwired: 3 in, 2 out]
    n280 = Unbundle By Name(w832) -> ("X Position"=→"X":sgl, "Y Position"=→"Y":sgl)
  }
  n281 = while {
    tunnel: w14 -> [w834]
    stop <- w833 stop-if-true
    n282 = Wait on Notification(notifier=w834) -> (notification=w836:T18, error out=w833:errorcluster)  [unwired: 3 in, 2 out]
    n283 = Unbundle By Name(w836) -> ("PiezoPosition"=→"PiezoPosition":sgl)
  }
  n284 = while {
    tunnel: w1 -> [w838]
    stop <- w840 stop-if-true
    n285 = Wait on Notification(notifier=w838) -> (notification=w839:T19, error out=w840:errorcluster)  [unwired: 3 in, 2 out]
    n286 = Unbundle By Name(w839) -> ("Readout"=→"Cap Readout":sgl)
  }
  n287 = Unregister For Events(event registration refnum=w27, error in=w34) -> (error out=w28:errorcluster)
  n288 = Merge Errors(w28, w35, w2) -> (w33:errorcluster)
  n289 = call "Destroy User Event - Stop.vi"("error in (no error)"=w33, "User Event - Stop"=w31) -> ("error out"=w21:errorcluster)  [unwired: 9 in]
  n290 = disable-structure shown="Default" {
    disable-tunnel: w21 -> [_ _]
    frame condition #0 {
      # "Call Quit LabVIEW if running as a built application."
      n291 = Quit LabVIEW() -> ()  [unwired: 1 in]
    }
    frame condition #1 (active) {
    }
  }
